vi "插入数据.vi"(5 "data":variant, 7 "columns":string[](array[string]), 8 "error in (no error)":errorcluster, 10 "database":string, 11 "table":string) -> (0 "error out":errorcluster)   [LabVIEW 2016, in "斯坦道总磷总氮.lvlib"]
uses:
  <vilib>/Utility/sysdir.llb/System Directory Type.ctl
  <vilib>/addons/database/Auxilliary.llb/DB Tools Transaction.ctl
  <vilib>/addons/database/Auxilliary.llb/DB Tools Isolation Level.ctl
  <vilib>/addons/database/Connection.llb/DB Tools Open Connec (String).vi
  <vilib>/addons/database/Connection.llb/Conn Transaction.vi
  <vilib>/addons/database/NI_Database_API.lvlib
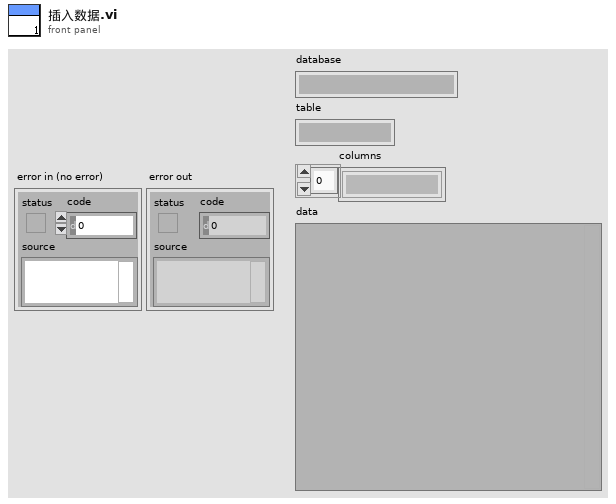
[diagram p1: front panel]
types:
  T1 = typedef "NI_Database_API.lvlib/DB Tools Transaction.ctl" = enum16{"begin", "commit", "rollback"}
  T2 = typedef "NI_Database_API.lvlib/DB Tools Isolation Level.ctl" = enum16{"chaos", "read uncommitted", "read committed", "repeatable read", "serializable"}
  T3 = typedef "System Directory Type.ctl" = i32
  T4 = typedef "NI_Database_API.lvlib/Conn ObjectReference.ctl" = refnum<k1>
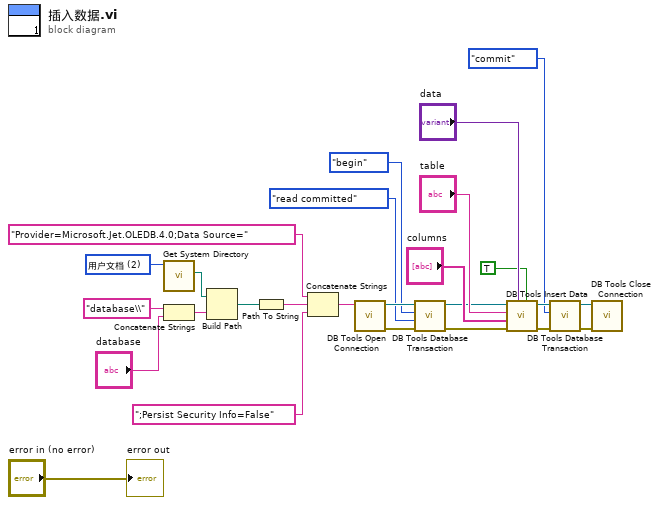
[diagram p0: block diagram]
diagram:
  w22 = T3 2 items=["用户目录"=0, "用户桌面"=1, "用户文档"=2, "用户应用程序数据"=3, "用户设置"=4, "用户临时目录"=5, "公共文档"=6, "公共应用程序数据"=7, "公共设置"=8, "公共缓存"=13, "系统核心库"=9, "系统安装库"=10, "应用程序文件"=11, "启动盘根目录"=12] ("system directory type")
  n1 = call <vilib>:"Get System Directory.vi"("system directory type"=w22) -> ("system directory"=w20:path)  [unwired: 10 in]
  n2 = Concatenate Strings("database\\" ("condition"), "database") -> (w14:string)
  n3 = Build Path(base path=w20, name or relative path=w14) -> (appended path=w19:path)
  n4 = Path To String(path=w19) -> (string=w18:string)
  n5 = Concatenate Strings("Provider=Microsoft.Jet.OLEDB.4.0;Data Source=" ("condition"), w18, ";Persist Security Info=False" ("condition")) -> (w16:string)
  n6 = call-poly <vilib>:"DB Tools Open Connection.vi"("connection information"=w16) -> ("error out"=w7:errorcluster, "connection reference"=w11:T4)  [unwired: 7 in]
  n7 = call-poly <vilib>:"DB Tools Database Transaction.vi"("error in (no error)"=w7, "isolation level (chaos)"=DB_Tools_Isolation_Level."read committed", "operation (begin)"=DB_Tools_Transaction."begin", "connection reference"=w11) -> ("error out"=w6:errorcluster, "connection reference out"=w9:T4)  [unwired: 2 in]
  n8 = call <vilib>:"DB Tools Insert Data.vi"("create table? (F)"=TRUE, "data"="data", "error in (no error)"=w6, "columns"="columns", "table"="table", "connection reference"=w9) -> ("error out"=w5:errorcluster, "connection reference out"=w26:T4)  [unwired: 4 in]
  n9 = call-poly <vilib>:"DB Tools Database Transaction.vi"("error in (no error)"=w5, "operation (begin)"=DB_Tools_Transaction."commit", "connection reference"=w26) -> ("error out"=w4:errorcluster, "connection reference out"=w8:T4)  [unwired: 3 in]
  n10 = call <vilib>:"DB Tools Close Connection.vi"("error in (no error)"=w4, "connection reference"=w8) -> ()  [unwired: 5 in, 1 out]
  "error out" <- "error in (no error)"
